vi "moveShutter.vi"(8 "error in (no error)":errorcluster, 10 "openingPercentage":T1=100.0 min=0.0 max=100.0, 11 "DomeController in":refnum<class "DomeController.lvclass">) -> (0 "error out":errorcluster, 3 "DomeController out":refnum<class "DomeController.lvclass">)   [LabVIEW 2016, in "DomeController.lvclass"]
uses:
  DomeController.lvclass
  IDome/domeTypedefs/openingPercentage.ctl
  domeCommunicator/ComTypedefs/commands.ctl
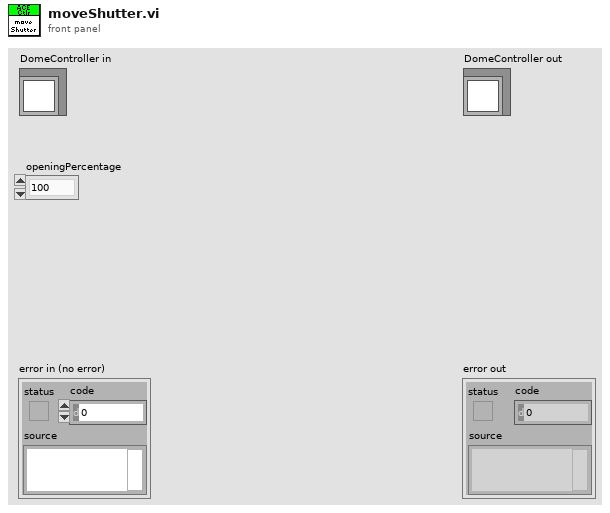
[diagram p1: front panel]
types:
  T1 = typedef "openingPercentage.ctl" = dbl
  T2 = typedef "commands.ctl" = enum16{"StopAllMotion", "CloseMainDoor", "OpenMainDoor", "CloseDropoutDoor", "OpenDropoutDoor", "SynchronizedOpen", "SynchronizedClose", "AutoShutDownOn", "AutoShutDownOff", "RainOn", "RainOff", "CloudSensorOn", "SloudSensorOff", "RotateToHomePosition", "MoveToAzimuth", "SetTolerance", "DefineHomePosition", "HighSpeedThreshold", "SetCoast", "SetEncoderCountFor360", "SetWatchDogTimer", "SetReverseDirectionMotionDelay", "SaveCurrentConfiguration"}
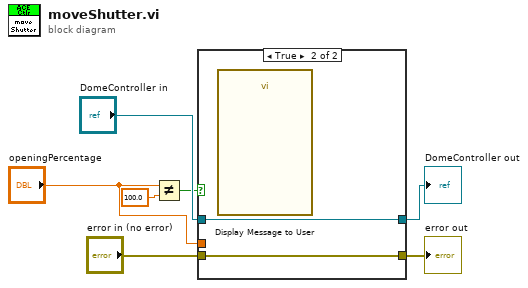
[diagram p0: block diagram]
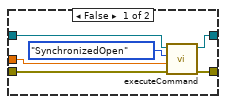
[diagram p2: hidden frame]
diagram:
  n1 = Not Equal?(x="openingPercentage", y=T1 100.0) -> (x != y?=w1:bool)
  n2 = case shown="True" w1 {
    tunnel: "DomeController in" -> [w13 w14]
    tunnel: [w12 w14] -> w6
    tunnel: "error in (no error)" -> [w11 w15]
    tunnel: [w10 w15] -> w4
    tunnel: "openingPercentage" -> [w8 _]
    frame False {
      n3 = call "executeCommand.vi"("error in (no error)"=w11, "Variant"=w8, "commands"=commands."SynchronizedOpen", "DomeController in"=w13) -> ("error out"=w10:errorcluster, "DomeController out"=w12:refnum<class "DomeController.lvclass">)  [unwired: 6 in]
    }
    frame True {
      n4 = call "Display Message to User"() -> ()  [unwired: 10 in, 2 out]
    }
  }
  "error out" <- w4
  "DomeController out" <- w6
